vi "设置窗口.vi"() -> ()   [LabVIEW 2016, in "仿真数据.lvlib"]
uses:
  <vilib>/Utility/config.llb/NI_LVConfig.lvlib
panel:
  in  "关闭时间":T1(ring)=enum."08"
  in  "开启时间":T2(ring)=enum."关闭"
  in  "关闭":bool
  in  "应用":bool
  in  "CODMN Reference data in":cluster{"参考数值":dbl[], "参考数值时间戳":timestamp[]}
  out "CODMN data in":cluster{"数值":dbl, "时间标识":timestamp}
  out "CODMN data out":T3
  in  "CODMN Para":T4 {"切换阈值" format="%#_6f"}
  in  "TN Reference data in":cluster{"参考数值":dbl[], "参考数值时间戳":timestamp[]}
  out "TN data in":cluster{"数值":dbl, "时间标识":timestamp}
  out "TN data out":T3
  in  "TN Para":T4 {"切换阈值" format="%#_6f"}
  in  "TP Reference data in":cluster{"参考数值":dbl[], "参考数值时间戳":timestamp[]}
  out "TP data in":cluster{"数值":dbl, "时间标识":timestamp}
  out "TP data out":T3
  in  "TP Para":T4 {"切换阈值" format="%#_6f"}
  in  "NH3N Reference data in":cluster{"参考数值":dbl[], "参考数值时间戳":timestamp[]}
  out "NH3N data in":cluster{"数值":dbl, "时间标识":timestamp}
  out "NH3N data out":T3
  in  "NH3N Para":T4 {"切换阈值" format="%#_6f"}
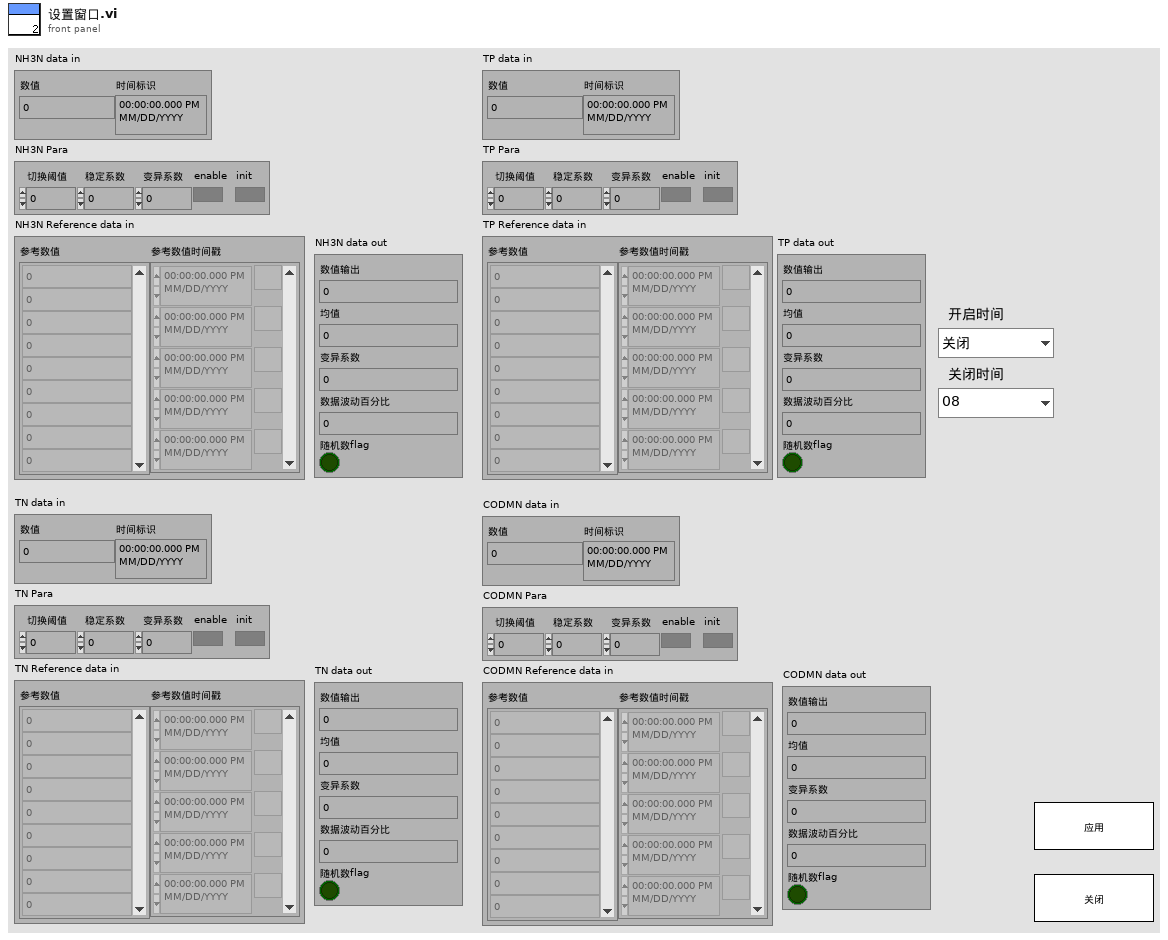
[diagram p1: front panel]
types:
  T1 = enum16{"00", "01", "02", "03", "04", "05", "06", "07", "08", "09", "10", "11", "12", "13", "14", "15", "16", "17", "18", "19", "20", "21", "22", "23"}
  T2 = enum16{"00", "01", "02", "03", "04", "05", "06", "07", "08", "09", "10", "11", "12", "13", "14", "15", "16", "17", "18", "19", "20", "21", "22", "23", "关闭"}
  T3 = cluster{"数值输出":dbl, "均值":dbl, "变异系数":dbl, "数据波动百分比":dbl, "随机数flag":bool}
  T4 = cluster{"切换阈值":dbl, "稳定系数":dbl, "变异系数":dbl, "enable":bool, "init":bool}
  T5 = typedef "NI_LVConfig.lvlib/Config Data RefNum.ctl" = refnum<k1>
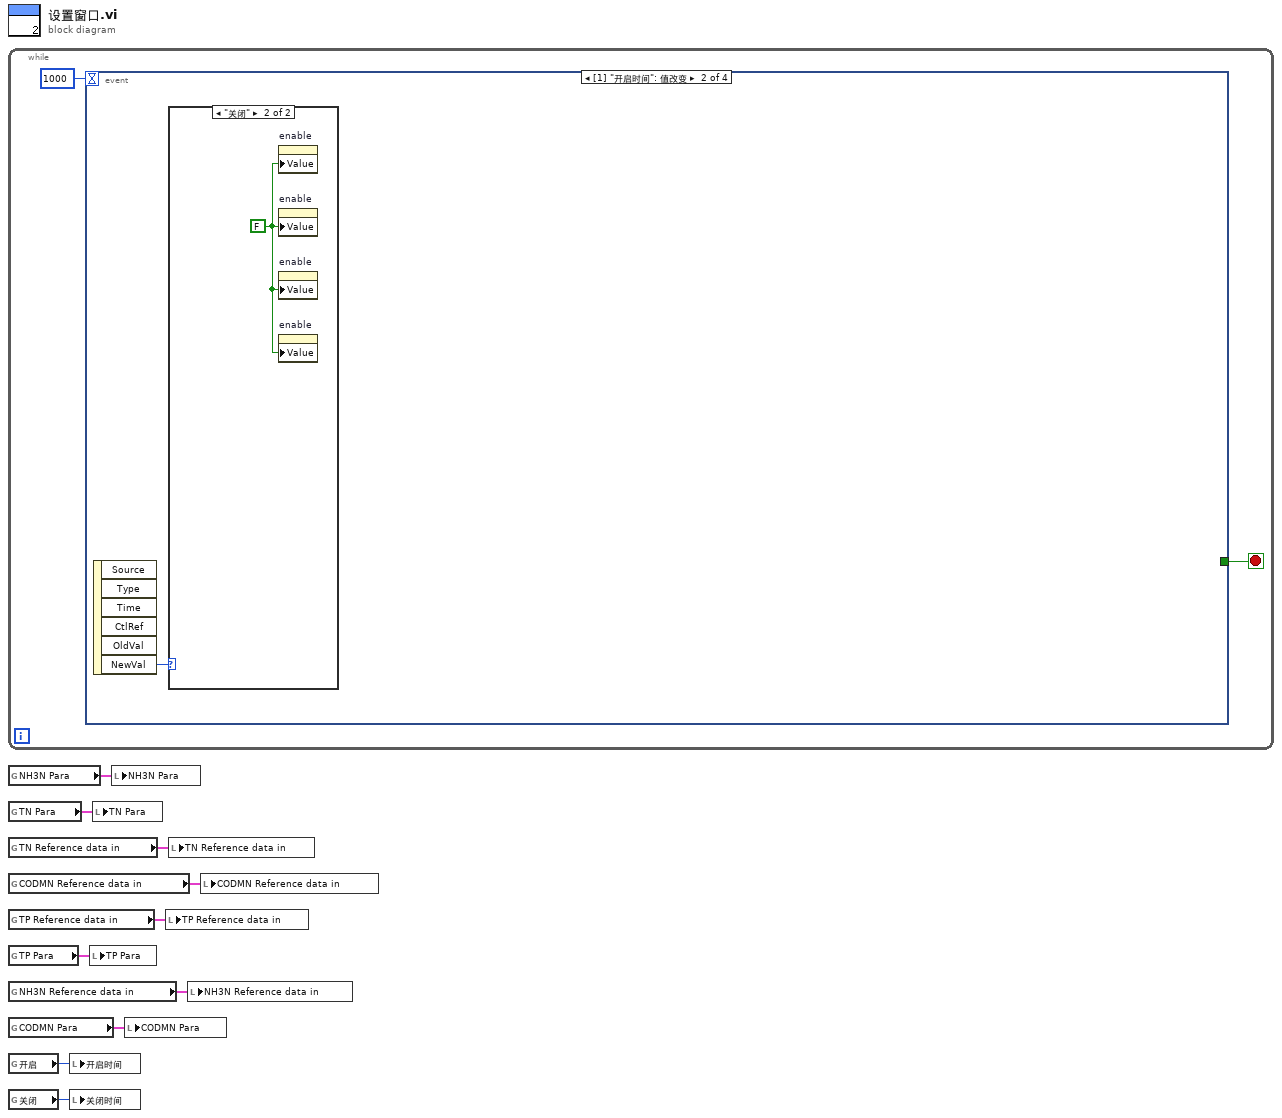
[diagram p0: block diagram]
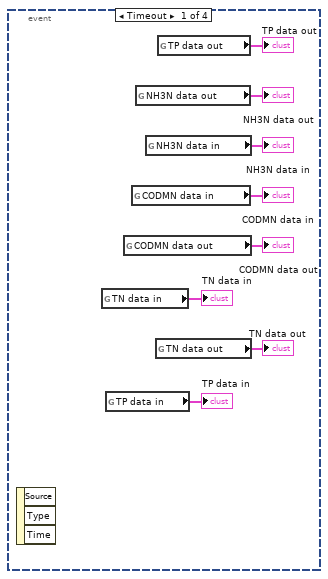
[diagram p2: hidden frame]
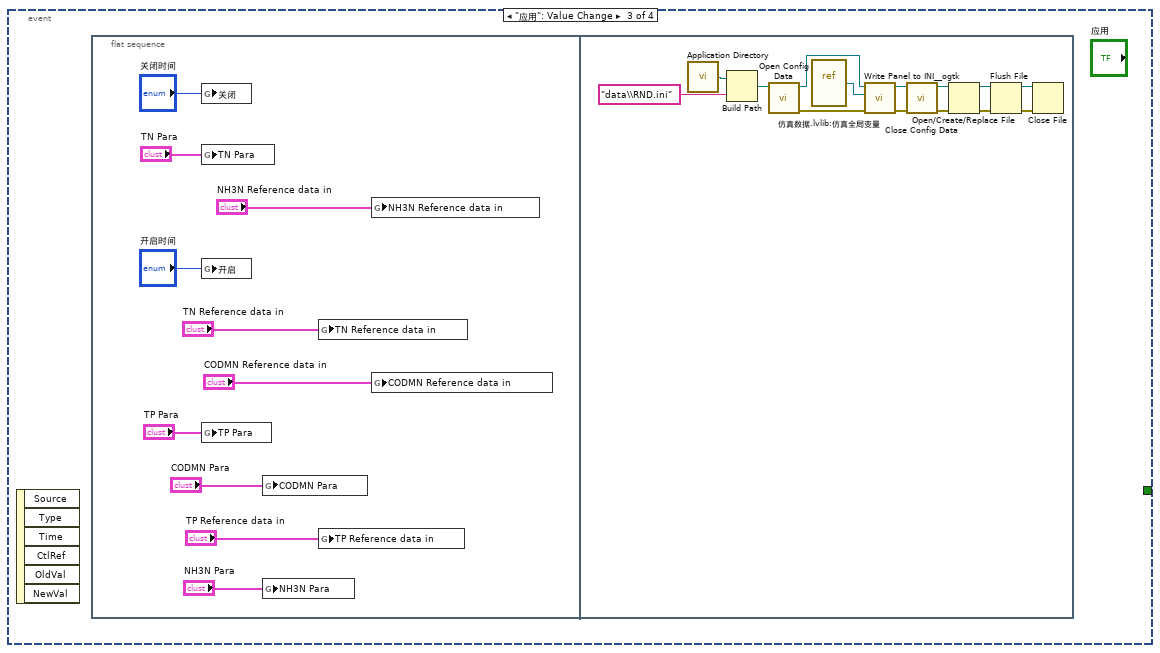
[diagram p4: hidden frame]
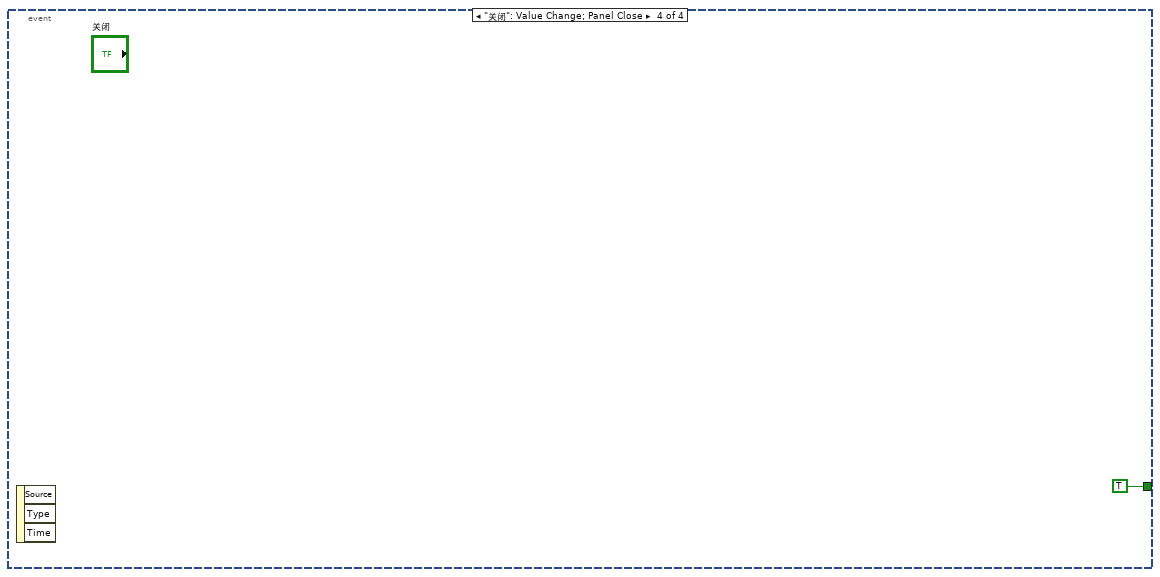
[diagram p5: hidden frame]
diagram:
  n1 = while {
    stop <- w12 stop-if-true
    n2 = event shown="[1] \"开启时间\": 值改变" {
      selector: _ -> [_ _ _ _]
      dyn-events: _ -> [_ _ _ _]
      timeout: 1000 -> [_ _ _ _]
      tunnel: [_ _ _ TRUE] -> w12
      event Timeout {
        n3 = event-data() -> ()  [unwired: 1 in, 3 out]
        n4 = global read "仿真全局变量.vi" "TN data in"() -> (→"TN data in":cluster{"数值":dbl, "时间标识":timestamp})
        n5 = global read "仿真全局变量.vi" "TP data in"() -> (→"TP data in":cluster{"数值":dbl, "时间标识":timestamp})
        n6 = global read "仿真全局变量.vi" "CODMN data out"() -> (→"CODMN data out":T3)
        n7 = global read "仿真全局变量.vi" "CODMN data in"() -> (→"CODMN data in":cluster{"数值":dbl, "时间标识":timestamp})
        n8 = global read "仿真全局变量.vi" "NH3N data out"() -> (→"NH3N data out":T3)
        n9 = global read "仿真全局变量.vi" "NH3N data in"() -> (→"NH3N data in":cluster{"数值":dbl, "时间标识":timestamp})
        n10 = global read "仿真全局变量.vi" "TN data out"() -> (→"TN data out":T3)
        n11 = global read "仿真全局变量.vi" "TP data out"() -> (→"TP data out":T3)
      }
      event "开启时间": Value Change {
        n12 = event-data() -> ("NewVal"=w21:T2)  [unwired: 1 in, 5 out]
        n13 = case shown="\"关闭\"" w21 {
          frame "00", Default {
          }
          frame "关闭" {
            w22 = FALSE
            n14 = property on="enable" class="Bool (严格)"("Value"=w22) -> ()  [unwired: 2 in, 2 out]
            n15 = property on="enable" class="Bool (严格)"("Value"=w22) -> ()  [unwired: 2 in, 2 out]
            n16 = property on="enable" class="Bool (严格)"("Value"=w22) -> ()  [unwired: 2 in, 2 out]
            n17 = property on="enable" class="Bool (严格)"("Value"=w22) -> ()  [unwired: 2 in, 2 out]
          }
        }
      }
      event "应用": Value Change {
        n18 = event-data() -> ()  [unwired: 1 in, 6 out]
        n19 = flat-sequence {
          frame #0 {
            n20 = global write "仿真全局变量.vi" "关闭"("关闭时间") -> ()
            n21 = global write "仿真全局变量.vi" "TN Para"("TN Para") -> ()
            n22 = global write "仿真全局变量.vi" "开启"("开启时间") -> ()
            n23 = global write "仿真全局变量.vi" "TP Para"("TP Para") -> ()
            n24 = global write "仿真全局变量.vi" "CODMN Para"("CODMN Para") -> ()
            n25 = global write "仿真全局变量.vi" "NH3N Para"("NH3N Para") -> ()
            n26 = global write "仿真全局变量.vi" "TN Reference data in"("TN Reference data in") -> ()
            n27 = global write "仿真全局变量.vi" "TP Reference data in"("TP Reference data in") -> ()
            n28 = global write "仿真全局变量.vi" "NH3N Reference data in"("NH3N Reference data in") -> ()
            n29 = global write "仿真全局变量.vi" "CODMN Reference data in"("CODMN Reference data in") -> ()
          }
          frame #1 {
            n30 = call <vilib>:"Application Directory.vi"() -> ("Application Directory"=w46:path)
            n31 = Build Path(base path=w46, name or relative path="data\\RND.ini" ("名称或相对路径")) -> (appended path=w44:path)
            n32 = call <vilib>:"Open Config Data.vi"("configuration file path"=w44) -> ("error out"=w40:errorcluster, "refnum"=w43:T5)  [unwired: 8 in, 1 out]
            n33 = vi-ref "仿真数据.lvlib:仿真全局变量.vi"() -> (w42:refnum<vi>)
            n34 = call <userlib>:"Write Panel to INI__ogtk.vi"("error in (no error)"=w40, "VI ref"=w42, "refnum"=w43) -> ("error out"=w39:errorcluster, "refnum out"=w41:T5)  [unwired: 7 in]
            n35 = call <vilib>:"Close Config Data.vi"("error in (no error)"=w39, "refnum"=w41) -> ("error out"=w34:errorcluster, "file path"=w33:path)  [unwired: 8 in]
            n36 = Open/Create/Replace File(file path (use dialog)=w33, error in=w34) -> (refnum out=w37:refnum<file>, error out=w38:errorcluster)  [unwired: 4 in, 1 out]
            n37 = Flush File(refnum=w37, error in=w38) -> (refnum out=w36:refnum<file>, error out=w35:errorcluster)
            n38 = Close File(refnum=w36, error in=w35) -> ()  [unwired: 2 out]
          }
        }
      }
      event "关闭": Value Change; Panel Close {
        n39 = event-data() -> ()  [unwired: 1 in, 3 out]
      }
    }
  }
  n40 = global read "仿真全局变量.vi" "NH3N Para"() -> (w9:T4)
  n41 = global read "仿真全局变量.vi" "TN Para"() -> (w7:T4)
  n42 = global read "仿真全局变量.vi" "TN Reference data in"() -> (w8:cluster{"参考数值":dbl[], "参考数值时间戳":timestamp[]})
  n43 = global read "仿真全局变量.vi" "CODMN Reference data in"() -> (w10:cluster{"参考数值":dbl[], "参考数值时间戳":timestamp[]})
  n44 = global read "仿真全局变量.vi" "TP Reference data in"() -> (w5:cluster{"参考数值":dbl[], "参考数值时间戳":timestamp[]})
  n45 = global read "仿真全局变量.vi" "TP Para"() -> (w3:T4)
  n46 = global read "仿真全局变量.vi" "NH3N Reference data in"() -> (w4:cluster{"参考数值":dbl[], "参考数值时间戳":timestamp[]})
  n47 = global read "仿真全局变量.vi" "CODMN Para"() -> (w6:T4)
  n48 = global read "仿真全局变量.vi" "开启"() -> (w2:T2)
  n49 = global read "仿真全局变量.vi" "关闭"() -> (w1:T1)
  n50 = local write "开启时间"(w2) -> ()
  n51 = local write "关闭时间"(w1) -> ()
  n52 = local write "TP Para"(w3) -> ()
  n53 = local write "TN Para"(w7) -> ()
  n54 = local write "NH3N Para"(w9) -> ()
  n55 = local write "CODMN Para"(w6) -> ()
  n56 = local write "TP Reference data in"(w5) -> ()
  n57 = local write "TN Reference data in"(w8) -> ()
  n58 = local write "NH3N Reference data in"(w4) -> ()
  n59 = local write "CODMN Reference data in"(w10) -> ()
